vi "Field Draw Path.vi"(0 "Pontos Smooth":dbl[][](array[numeric]), 1 "function":T1, 4 "Lado":enum16{"Esquerdo", "Direito"}(ring) caption="Enum", 6 "Draw Targets?":T3, 8 "Scale mm/pixel":dbl, 9 "Offset":T4, 10 "Pontos":dbl[][](array[numeric]), 11 "picture in":picture) -> (2 "picture out":picture)   [LabVIEW 2017]
uses:
  <vilib>/Utility/miscctls.llb/LVBoundsTypeDef.ctl
  DrawTargets.ctl
  Intel/Functions Enum.ctl
panel:
  in  "pen 2":T2={"Width"=3, "Style"=enum."Solid"}
  in  "pen":T2={"Width"=3, "Style"=enum."Solid"}
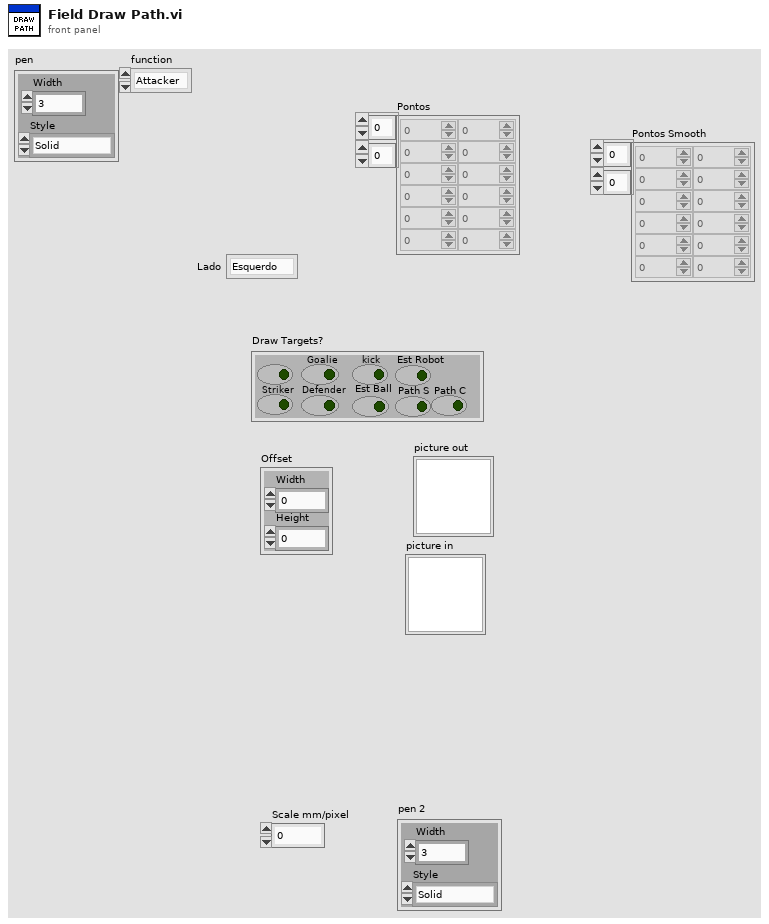
[diagram p1: front panel]
types:
  T1 = typedef "Functions Enum.ctl" = enum16{"Attacker", "Goalie", "Defender", "Striker", "Goto 0", "Dummy", "Kicker", "ZigZag"}
  T2 = cluster{"Width":u16, "Style":enum32{"Solid", "Dash", "Dot", "DashDot", "DashDotDot"}}
  T3 = typedef "DrawTargets.ctl" = cluster{"Attacker":bool, "Striker":bool, "Goalie":bool, "Defender":bool, "kick":bool, "Est Ball":bool, "Est Robot":bool, "Path S":bool, "Path C":bool}
  T4 = typedef "LVBoundsTypeDef.ctl" = cluster{"Width":u32, "Height":u32}
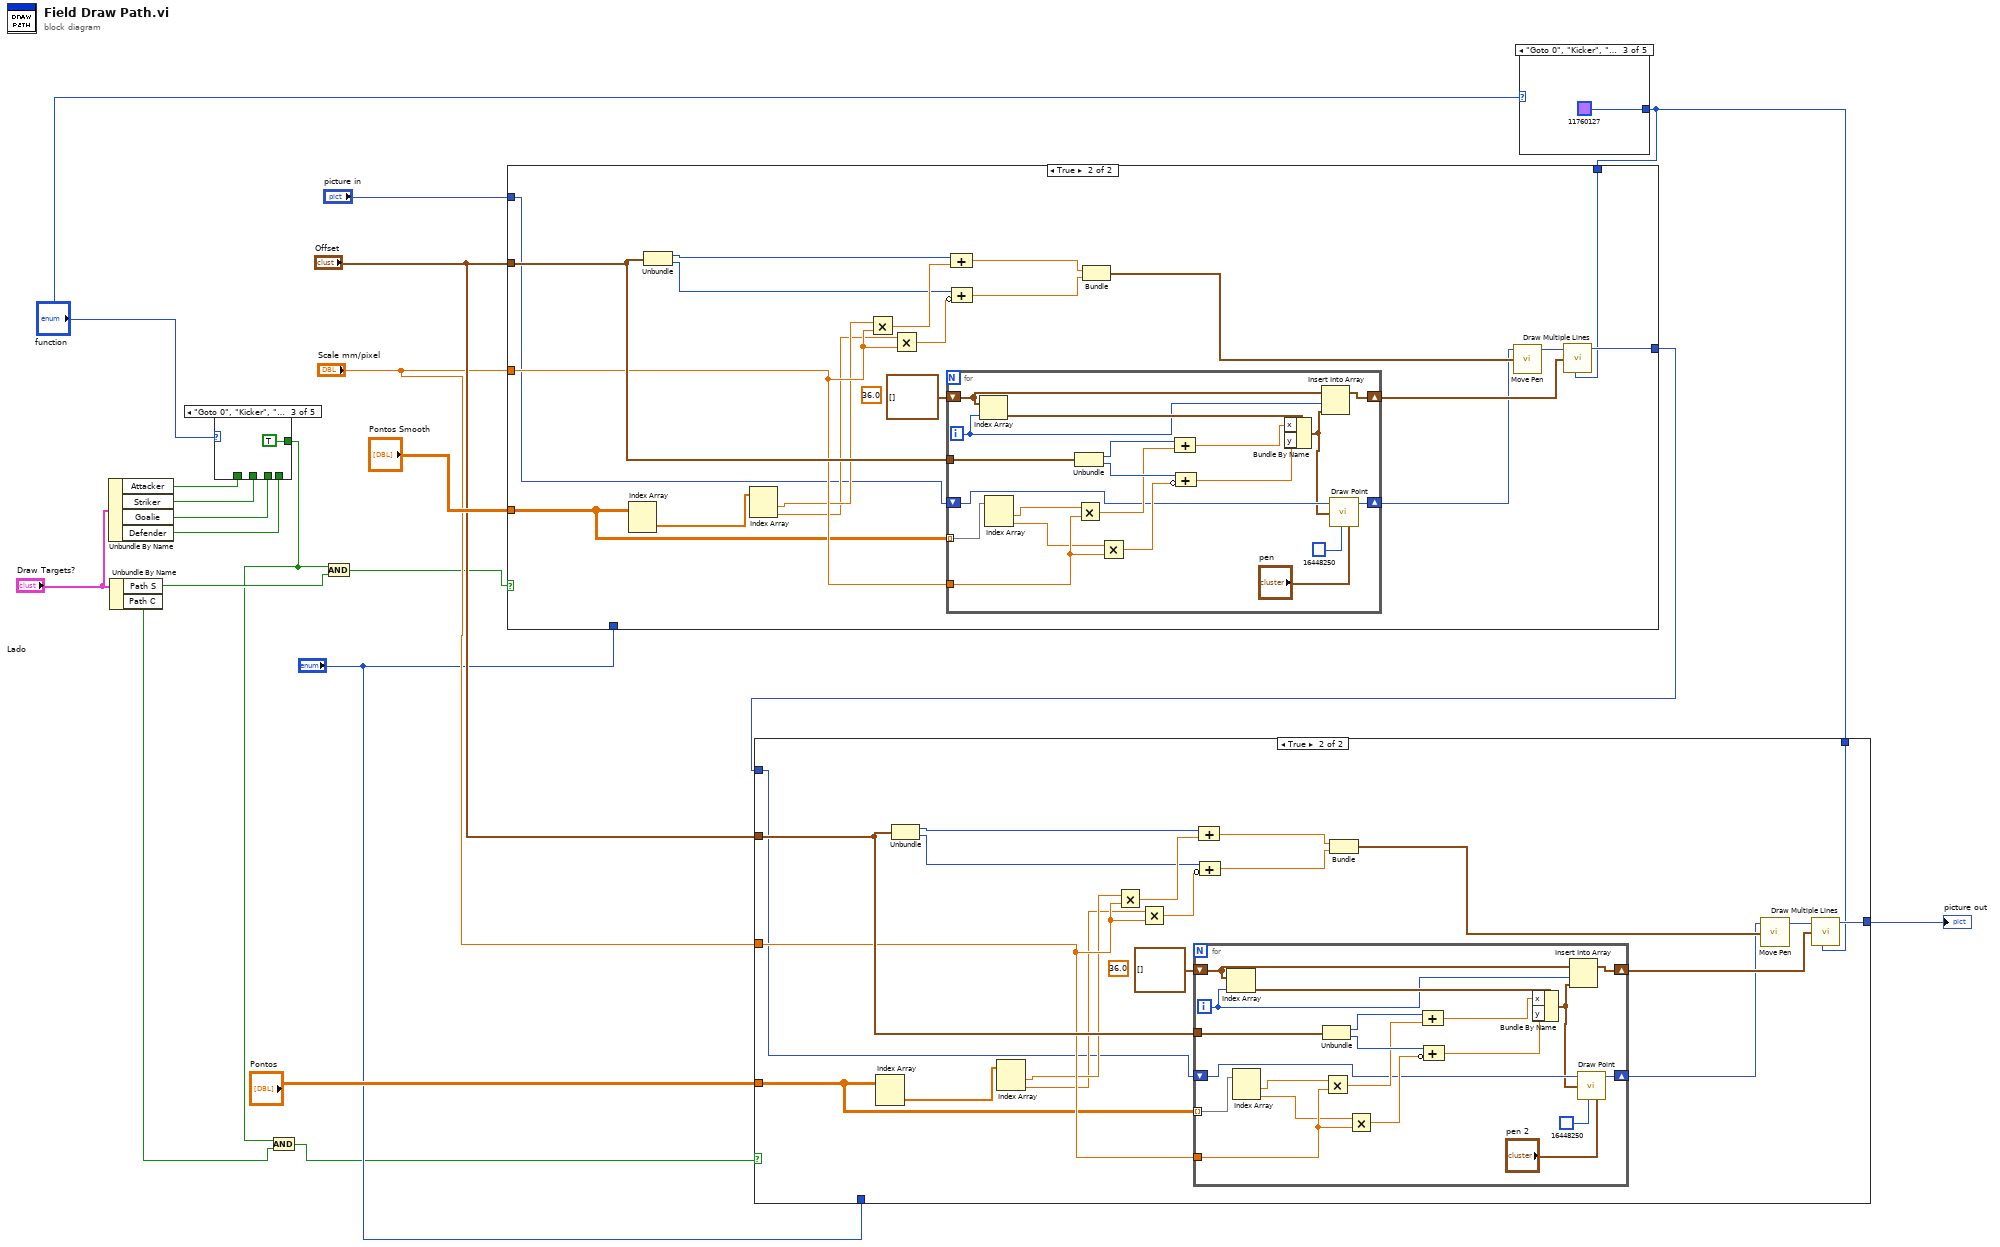
[diagram p0: block diagram]
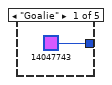
[diagram p6: hidden frame]
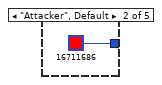
[diagram p7: hidden frame]
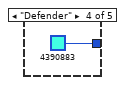
[diagram p8: hidden frame]
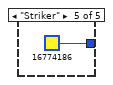
[diagram p9: hidden frame]
diagram:
  n1 = Unbundle By Name("Draw Targets?") -> ("Attacker"=w9:bool, "Striker"=w10:bool, "Goalie"=w8:bool, "Defender"=w11:bool)
  n2 = Unbundle By Name("Draw Targets?") -> ("Path S"=w4:bool, "Path C"=w2:bool)
  n3 = case shown="\"Goto 0\", \"Kicker\", \"ZigZag\"" "function" {
    tunnel: [w21 w22 TRUE ("Draw Target Striker?") w24 w25] -> w3
    tunnel: w11 -> [_ _ _ w24 _]
    tunnel: w10 -> [_ _ _ _ w25]
    tunnel: w9 -> [w21 _ _ _ _]
    tunnel: w8 -> [_ w22 _ _ _]
    frame "Attacker", Default {
    }
    frame "Goalie" {
    }
    frame "Goto 0", "Kicker", "ZigZag" {
    }
    frame "Defender" {
    }
    frame "Striker" {
    }
  }
  n4 = And(x=w3, y=w2) -> (x .and. y?=w1:bool)
  n5 = And(x=w3, y=w4) -> (x .and. y?=w5:bool)
  n6 = case shown="\"Goto 0\", \"Kicker\", \"ZigZag\"" "function" {
    tunnel: [u32 14047743 ("color(black)") u32 16711686 ("color(black)") u32 11760127 ("color(black)") u32 4390883 ("color(black)") u32 16774186 ("color(black)")] -> w12
    frame "Goalie" {
    }
    frame "Attacker", Default {
    }
    frame "Goto 0", "Kicker", "ZigZag" {
    }
    frame "Defender" {
    }
    frame "Striker" {
    }
  }
  n7 = case shown="True" w5 {
    tunnel: [w31 w33] -> w18
    tunnel: "Offset" -> [_ w44]
    tunnel: "Scale mm/pixel" -> [_ w43]
    tunnel: "picture in" -> [w31 w35]
    tunnel: "Lado" -> [_ _]
    tunnel: "Pontos Smooth" -> [_ w38]
    tunnel: w12 -> [_ w32]
    frame False {
    }
    frame True {
      (unwired) sgl 36.0 ("radius")
      n8 = Index Array(array=w38) -> (element=w41:dbl[])  [unwired: 2 in]
      n9 = Unbundle(w44) -> ("Width"=w51:u32, "Height"=w48:u32)
      n10 = Index Array(array=w41) -> (element #1=w40:dbl, element #2=w39:dbl)  [unwired: 2 in]
      n11 = Multiply(x=w40, y=w43) -> (x*y=w50:dbl)
      n12 = Multiply(x=w39, y=w43) -> (x*y=w47:dbl)
      n13 = for {
        tunnel: w44 -> [w69]
        tunnel: w43 -> [w68]
        tunnel: w38 -> [w65] mode=indexing
        shift-right: [w57] -> w36
        shift-left: cluster{"x":i16, "y":i16}[] [] ("line endpoints") -> [w58]
        shift-right: [w55] -> w34
        shift-left: w35 -> [w56]
        i -> [w59]
        n14 = Index Array(array=w58, index=w59) -> (element=w60:cluster{"x":i16, "y":i16})
        n15 = Index Array(array=w65) -> (element #1=w64:dbl, element #2=w63:dbl)  [unwired: 2 in]
        n16 = Unbundle(w69) -> ("Width"=w71:u32, "Height"=w70:u32)
        n17 = Multiply(x=w64, y=w68) -> (x*y=w67:dbl)
        n18 = Multiply(x=w63, y=w68) -> (x*y=w66:dbl)
        n19 = Compound Arithmetic op=ADD(w71, w67) -> (w62:dbl)
        n20 = Compound Arithmetic op=ADD(w70, invert w66) -> (w61:dbl)
        n21 = Bundle By Name(cluster=w60, "x"=w62, "y"=w61) -> (w53:cluster{"x":i16, "y":i16})
        n22 = Insert Into Array(array=w58, index=w59, new element=w53) -> (w57:cluster{"x":i16, "y":i16}[])
        n23 = call <vilib>:"Draw Point.vi"("picture"=w56, "point(x,y)"=w53, "color(black)"=u32 16448250, "pen"="pen") -> ("new picture"=w55:picture)  [unwired: 5 in]
      }
      n24 = Compound Arithmetic op=ADD(w51, w50) -> (w49:dbl)
      n25 = Compound Arithmetic op=ADD(w48, invert w47) -> (w46:dbl)
      n26 = Bundle(w49, w46) -> (w42:cluster{dbl, dbl})  [unwired: 1 in]
      n27 = call <vilib>:"Move Pen.vi"("new position"=w42, "picture"=w34) -> ("new picture"=w45:picture)  [unwired: 3 in]
      n28 = call <vilib>:"Draw Multiple Lines.vi"("picture"=w45, "line endpoints"=w36, "color(black)"=w32) -> ("new picture"=w33:picture)  [unwired: 6 in]
    }
  }
  n29 = case shown="True" w1 {
    tunnel: [w72 w74] -> w13
    tunnel: "Offset" -> [_ w85]
    tunnel: "Scale mm/pixel" -> [_ w84]
    tunnel: w18 -> [w72 w76]
    tunnel: "Lado" -> [_ _]
    tunnel: "Pontos" -> [_ w79]
    tunnel: w12 -> [_ w73]
    frame False {
    }
    frame True {
      (unwired) sgl 36.0 ("radius")
      n30 = Index Array(array=w79) -> (element=w82:dbl[])  [unwired: 2 in]
      n31 = Unbundle(w85) -> ("Width"=w92:u32, "Height"=w89:u32)
      n32 = Index Array(array=w82) -> (element #1=w81:dbl, element #2=w80:dbl)  [unwired: 2 in]
      n33 = Multiply(x=w81, y=w84) -> (x*y=w91:dbl)
      n34 = Multiply(x=w80, y=w84) -> (x*y=w88:dbl)
      n35 = for {
        tunnel: w85 -> [w110]
        tunnel: w84 -> [w109]
        tunnel: w79 -> [w106] mode=indexing
        shift-right: [w98] -> w77
        shift-left: cluster{"x":i16, "y":i16}[] [] ("line endpoints") -> [w99]
        shift-right: [w96] -> w75
        shift-left: w76 -> [w97]
        i -> [w100]
        n36 = Index Array(array=w99, index=w100) -> (element=w101:cluster{"x":i16, "y":i16})
        n37 = Index Array(array=w106) -> (element #1=w105:dbl, element #2=w104:dbl)  [unwired: 2 in]
        n38 = Unbundle(w110) -> ("Width"=w112:u32, "Height"=w111:u32)
        n39 = Multiply(x=w105, y=w109) -> (x*y=w108:dbl)
        n40 = Multiply(x=w104, y=w109) -> (x*y=w107:dbl)
        n41 = Compound Arithmetic op=ADD(w112, w108) -> (w103:dbl)
        n42 = Compound Arithmetic op=ADD(w111, invert w107) -> (w102:dbl)
        n43 = Bundle By Name(cluster=w101, "x"=w103, "y"=w102) -> (w94:cluster{"x":i16, "y":i16})
        n44 = Insert Into Array(array=w99, index=w100, new element=w94) -> (w98:cluster{"x":i16, "y":i16}[])
        n45 = call <vilib>:"Draw Point.vi"("picture"=w97, "point(x,y)"=w94, "color(black)"=u32 16448250, "pen"="pen 2") -> ("new picture"=w96:picture)  [unwired: 5 in]
      }
      n46 = Compound Arithmetic op=ADD(w92, w91) -> (w90:dbl)
      n47 = Compound Arithmetic op=ADD(w89, invert w88) -> (w87:dbl)
      n48 = Bundle(w90, w87) -> (w83:cluster{dbl, dbl})  [unwired: 1 in]
      n49 = call <vilib>:"Move Pen.vi"("new position"=w83, "picture"=w75) -> ("new picture"=w86:picture)  [unwired: 3 in]
      n50 = call <vilib>:"Draw Multiple Lines.vi"("picture"=w86, "line endpoints"=w77, "color(black)"=w73) -> ("new picture"=w74:picture)  [unwired: 6 in]
    }
  }
  "picture out" <- w13
